vi "Trim instances for uniques.vi"(0 "Paper names":string[](array[string]), 1 "Undelivered instances in":T1[](array[typedef])) -> (2 "Undelivered instances out":T1[](array[typedef]))   [LabVIEW 2015]
uses:
  Home/Undelivered instance.ctl
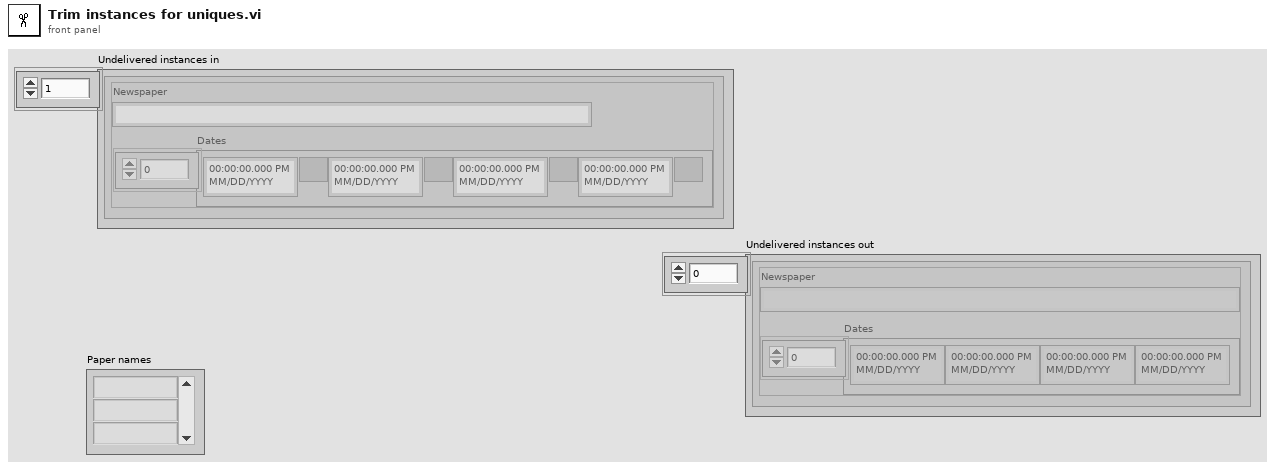
[diagram p1: front panel]
types:
  T1 = typedef "Undelivered instance.ctl" = cluster{"Dates":timestamp[], "Newspaper":string}
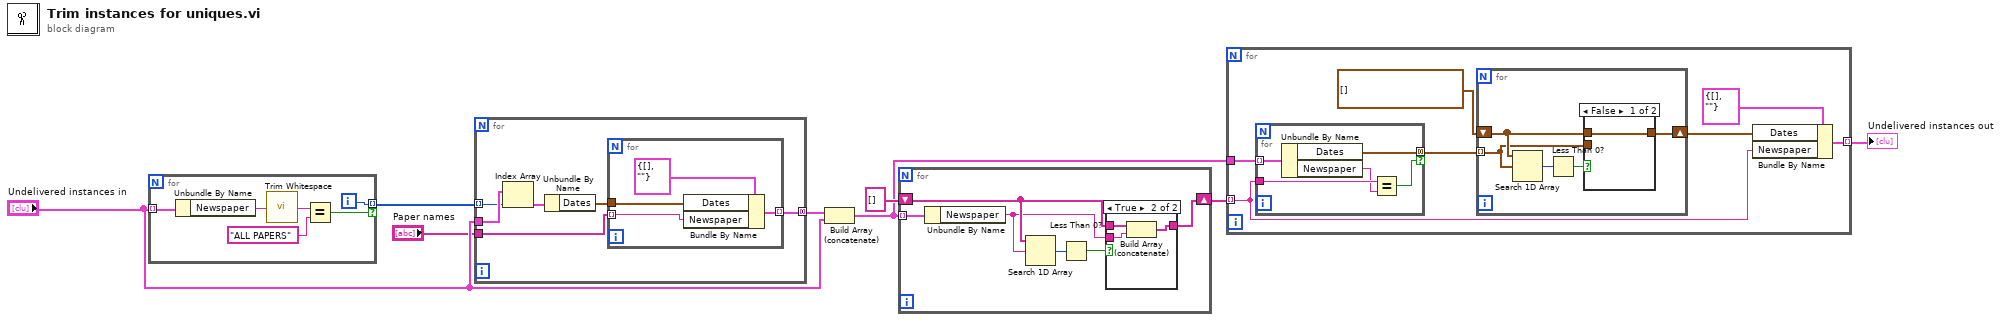
[diagram p0: block diagram]
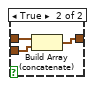
[diagram p2: hidden frame]
diagram:
  n1 = for {
    tunnel: "Undelivered instances in" -> [w14] mode=indexing
    tunnel: [w11] -> w4 mode=indexing if=w10
    i -> [w11]
    n2 = Unbundle By Name(w14) -> ("Newspaper"=w13:string)
    n3 = call <vilib>:"Trim Whitespace.vi"("string"=w13) -> ("trimmed string"=w9:string)  [unwired: 1 in]
    n4 = Equal?(x=w9, y="ALL PAPERS") -> (x = y?=w10:bool)
  }
  n5 = for {
    tunnel: w4 -> [w19] mode=indexing
    tunnel: "Undelivered instances in" -> [w20]
    tunnel: "Paper names" -> [w17]
    tunnel: [w15] -> w1 mode=concatenating
    n6 = Index Array(array=w20, index=w19) -> (element=w18:T1)
    n7 = Unbundle By Name(w18) -> ("Dates"=w16:timestamp[])
    n8 = for {
      tunnel: w17 -> [w23] mode=indexing
      tunnel: w16 -> [w22]
      tunnel: [w21] -> w15 mode=indexing
      n9 = Bundle By Name(cluster=T1 {"Dates"=[], "Newspaper"=""} ("Paper instance"), "Dates"=w22, "Newspaper"=w23) -> (w21:T1)
    }
  }
  n10 = Build Array (concatenate)(w1, "Undelivered instances in") -> (w5:T1[])
  n11 = for {
    tunnel: w5 -> [w30] mode=indexing
    shift-right: [w29] -> w7
    shift-left: string[] [] -> [w28]
    n12 = Unbundle By Name(w30) -> ("Newspaper"=w27:string)
    n13 = Search 1D Array(1D array=w28, element=w27) -> (index of element=w26:i32)  [unwired: 1 in]
    n14 = Less Than 0?(x=w26) -> (x < 0?=w25:bool)
    n15 = case shown="True" w25 {
      tunnel: w27 -> [_ w34]
      tunnel: w28 -> [w31 w33]
      tunnel: [w31 w32] -> w29
      frame False {
      }
      frame True {
        n16 = Build Array (concatenate)(w33, w34) -> (w32:string[])
      }
    }
  }
  n17 = for {
    tunnel: w7 -> [w36] mode=indexing
    tunnel: w5 -> [w41]
    tunnel: [w35] -> w6 mode=indexing
    n18 = for {
      tunnel: w41 -> [w55] mode=indexing
      tunnel: w36 -> [w54]
      tunnel: [w51] -> w40 mode=concatenating if=w53
      n19 = Unbundle By Name(w55) -> ("Dates"=w51:timestamp[], "Newspaper"=w52:string)
      n20 = Equal?(x=w54, y=w52) -> (x = y?=w53:bool)
    }
    n21 = for {
      tunnel: w40 -> [w44] mode=indexing
      shift-right: [w46] -> w37
      shift-left: timestamp[] [] -> [w45]
      n22 = Search 1D Array(1D array=w45, element=w44) -> (index of element=w43:i32)  [unwired: 1 in]
      n23 = Less Than 0?(x=w43) -> (x < 0?=w42:bool)
      n24 = case shown="False" w42 {
        tunnel: w44 -> [_ w50]
        tunnel: w45 -> [w47 w49]
        tunnel: [w47 w48] -> w46
        frame False {
        }
        frame True {
          n25 = Build Array (concatenate)(w49, w50) -> (w48:timestamp[])
        }
      }
    }
    n26 = Bundle By Name(cluster=T1 {"Dates"=[], "Newspaper"=""} ("Paper instance"), "Dates"=w37, "Newspaper"=w36) -> (w35:T1)
  }
  "Undelivered instances out" <- w6
